vi "Get UI References.vi"(8 "error in (no error)":errorcluster, 11 "VI reference":refnum<vi>) -> (0 "error out":errorcluster, 3 "Controls[]":refnum<vi>[](array[refnum]))   [LabVIEW 2019, in "uiControlsMgr.lvclass"]
uses:
  uiControlsMgr.lvclass
panel:
  out "Array":errorcluster[](array[cluster])
  out "Table":string[][](table)
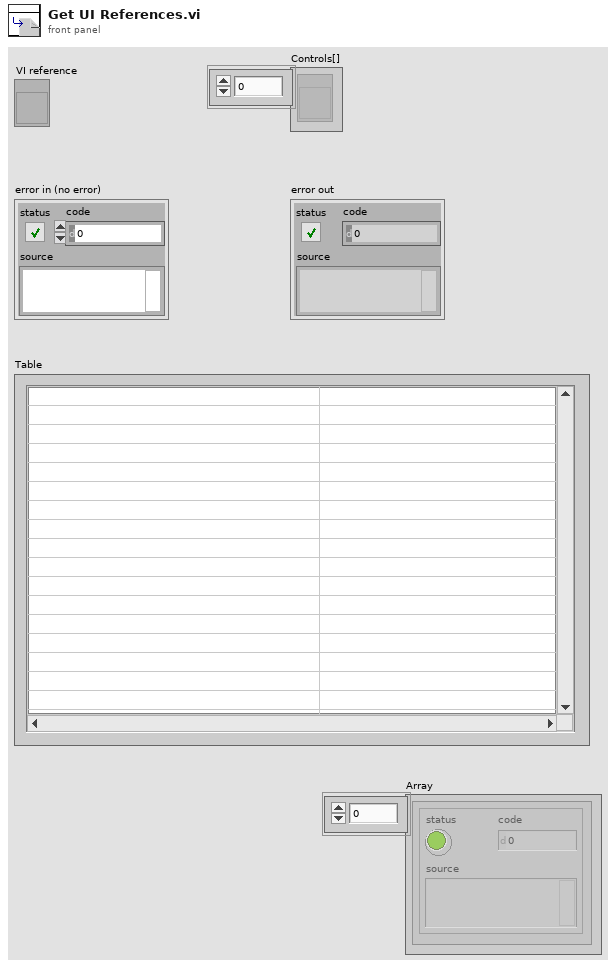
[diagram p1: front panel]
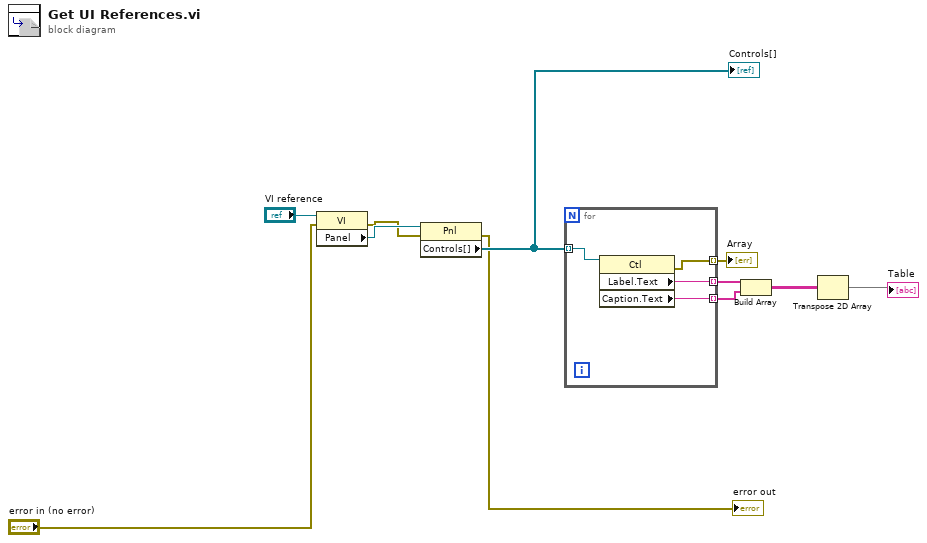
[diagram p0: block diagram]
diagram:
  n1 = property class="VI"(reference="VI reference", error in="error in (no error)") -> (error out=w4:errorcluster, "Panel"=w10:refnum<vi>)  [unwired: 1 out]
  n2 = property class="Pnl"(reference=w10, error in=w4) -> (error out=→"error out":errorcluster, "Controls[]"=w11:refnum<vi>[])  [unwired: 1 out]
  "Controls[]" <- w11
  n3 = for {
    tunnel: w11 -> [w13] mode=indexing
    tunnel: [w15] -> w9 mode=indexing
    tunnel: [w14] -> w8 mode=indexing
    tunnel: [w12] -> w1 mode=indexing
    n4 = property class="Ctl"(reference=w13) -> (error out=w12:errorcluster, "Label.Text"=w15:string, "Caption.Text"=w14:string)  [unwired: 1 in, 1 out]
  }
  "Array" <- w1
  n5 = Build Array(w9, w8) -> (w7:string[][])
  n6 = Transpose 2D Array(2D array=w7) -> (transposed array=→"Table":string[][])
